vi "StateSpaceUtil_ClampInputMaxMagnitude.vi"(9 "U_max":T1, 10 "U_min":T1, 11 "U":T1) -> (0 "Size Coerced":bool, 3 "ClampedU":T1)   [LabVIEW 2019, in "Trajectory_Library.lvlib"]
doc: "Clamp the input u to the min and max.\n \nInputs:\n - u -- The input to clamp.\n - umin -- The minimum input magnitude.\n - umax -- The maximum input magnitude.\n\nOutputs:\n - ClampedU -- The clamped input.\n - sizeCoerced -- If TRUE, an error occured."
uses:
  Trajectory_Library.lvlib
  <vilib>/Analysis/Matrix/Datatypes/RealMatrix.ctl
  <vilib>/Analysis/Matrix/NI_Matrix.lvlib
panel:
  # "<J ,1>"
  # "<J ,1>"
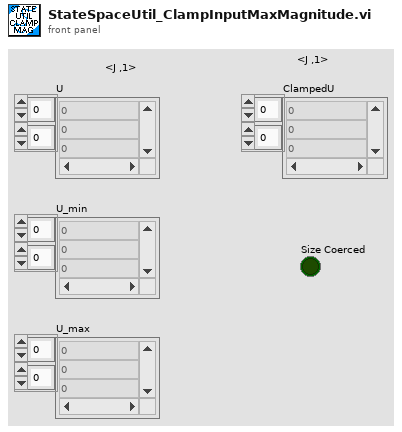
[diagram p1: front panel]
types:
  T1 = typedef "NI_Matrix.lvlib/RealMatrix.ctl" = dbl[][]
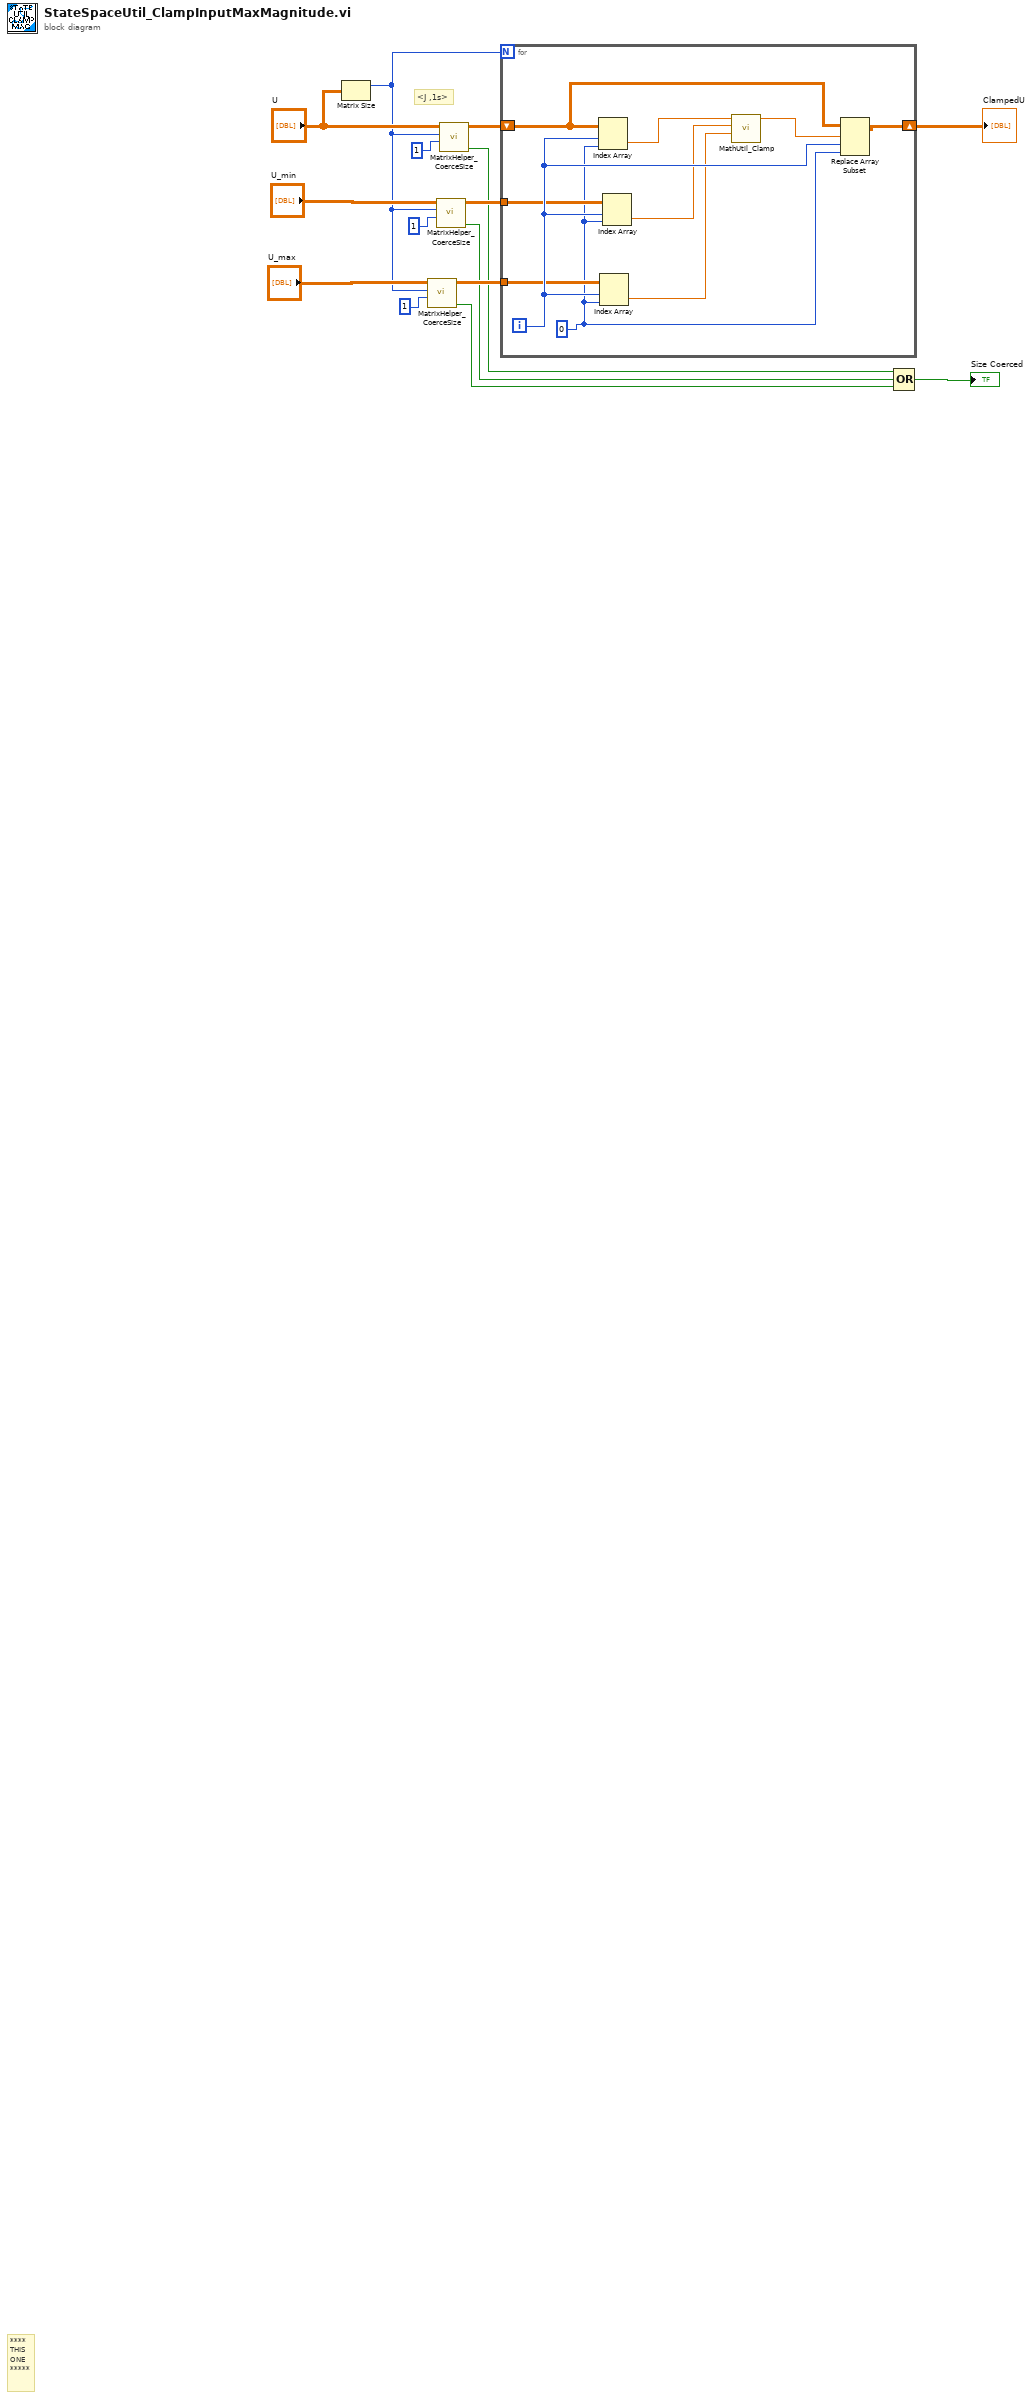
[diagram p0: block diagram]
diagram:
  # "<J ,1s>"
  # "****\nTHIS\nONE\n*****"
  n1 = Matrix Size(0:"U") -> (1:w9:i32)  [unwired: 1 out]
  n2 = call "MatrixHelper_CoerceSize.vi"("Columns"=1 ("number of columns"), "Rows"=w9, "input matrix"="U_max") -> ("Coerced"=w2:bool, "output matrix"=w6:T1)  [unwired: 7 in]
  n3 = call "MatrixHelper_CoerceSize.vi"("Columns"=1 ("number of columns"), "Rows"=w9, "input matrix"="U_min") -> ("Coerced"=w3:bool, "output matrix"=w7:T1)  [unwired: 7 in]
  n4 = call "MatrixHelper_CoerceSize.vi"("Columns"=1 ("number of columns"), "Rows"=w9, "input matrix"="U") -> ("Coerced"=w4:bool, "output matrix"=w8:T1)  [unwired: 7 in]
  n5 = for {
    N: w9 -> [_]
    tunnel: w7 -> [w24]
    tunnel: w6 -> [w23]
    shift-right: [w21] -> w5
    shift-left: w8 -> [w20]
    i -> [w25]
    w22 = 0 ("index (col)")
    n6 = Index Array(array=w20, index (row)=w25, index (col)=w22) -> (element=w18:dbl)
    n7 = Index Array(array=w23, index (row)=w25, index (col)=w22) -> (element=w16:dbl)
    n8 = Index Array(array=w24, index (row)=w25, index (col)=w22) -> (element=w17:dbl)
    n9 = call "MathUtil_Clamp.vi"("High Limit"=w16, "Low Limit"=w17, "Value"=w18) -> ("Result"=w19:dbl)  [unwired: 8 in]
    n10 = Replace Array Subset(array=w20, new element=w22, index (row)=w19, index (col)=w25) -> (w21:T1)
  }
  "ClampedU" <- w5
  n11 = Compound Arithmetic op=OR(w4, w3, w2) -> (→"Size Coerced":bool)
